vi "Decimal2(SubVI).vi"(11 "DC estimate (V)":dbl) -> (3 "Numeric":dbl)   [LabVIEW 2019]
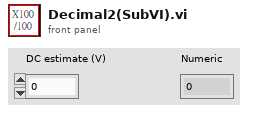
[diagram p1: front panel]
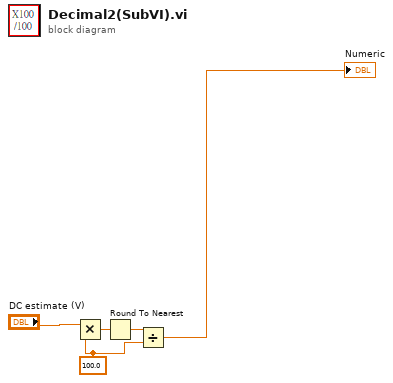
[diagram p0: block diagram]
diagram:
  w2 = 100.0 ("y")
  n1 = Multiply(x="DC estimate (V)", y=w2) -> (x*y=w1:dbl)
  n2 = Round To Nearest(number=w1) -> (nearest integer value=w3:dbl)
  n3 = Divide(x=w3, y=w2) -> (x/y=→"Numeric":dbl)
